vi "Block Function Item.vi"(11 "模块名称":string="测试工作站") -> (3 "模块定义":T1)   [LabVIEW 2018, in "MainInterface.lvlib"]
uses:
  MainInterface.lvlib
  ModuleInterface/ModuleDefinition.ctl
  ModuleInterface/FunctionItem.ctl
  ModuleInterface/ModuleInterface.lvlib
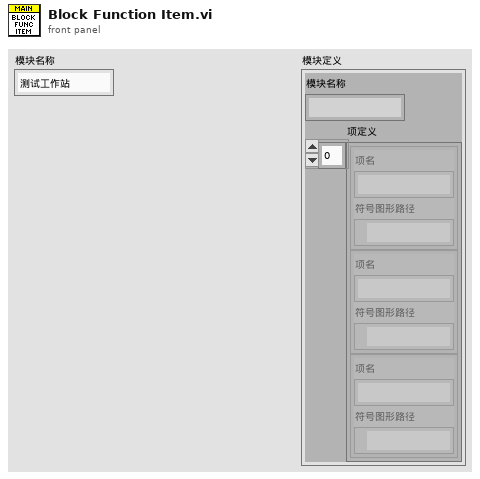
[diagram p1: front panel]
types:
  T1 = typedef "ModuleInterface.lvlib/ModuleDefinition.ctl" = cluster{"模块名称":string, "项定义":T2[]}
  T2 = typedef "ModuleInterface.lvlib/FunctionItem.ctl" = cluster{"项名":string, "符号图形路径":path}
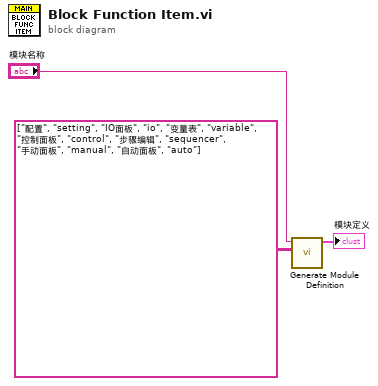
[diagram p0: block diagram]
diagram:
  n1 = call "Generate Module Definition.vi"("数组"=string[][] [["配置", "setting"], ["IO面板", "io"], ["变量表", "variable"], ["控制面板", "control"], ["步骤编辑", "sequencer"], ["手动面板", "manual"], ["自动面板", "auto"]], "模块名称"="模块名称") -> ("模块定义"=→"模块定义":T1)  [unwired: 9 in]
